vi "Tick Quadrature State.vi"(7 "Forward? (T)":bool=TRUE, 8 "error in (no error)":errorcluster, 9 "Current State":i32, 10 "Channels":string[](array[string])=[" ", ""], 11 "WorkspaceManager in":T1) -> (0 "error out":errorcluster, 1 "New State":i32, 3 "WorkspaceManager out":T1)   [LabVIEW 2026, in "Scan Engine Specialty Digital System Tests.lvclass"]
uses:
  Scan Engine Specialty Digital System Tests.lvclass
  <vilib>/NI/VeriStand Custom Device Testing Tools/VeriStandTestUtilities/VeriStandTestUtilities.lvlib
  <vilib>/NI VeriStand/Execution/Workspace/WorkspaceAPI.ctl
  <vilib>/NI VeriStand/Execution/Workspace/NI_VS Workspace ExecutionAPI.lvlib
  NationalInstruments.VeriStand.ClientAPI
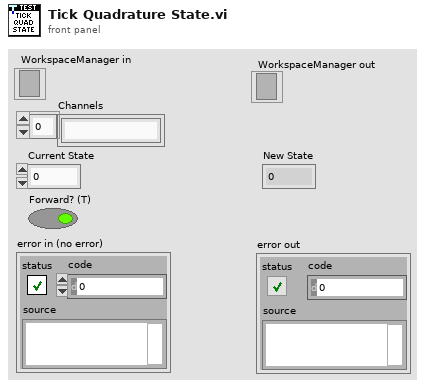
[diagram p1: front panel]
types:
  T1 = typedef "NI_VS Workspace ExecutionAPI.lvlib/WorkspaceAPI.ctl" = refnum<k24>
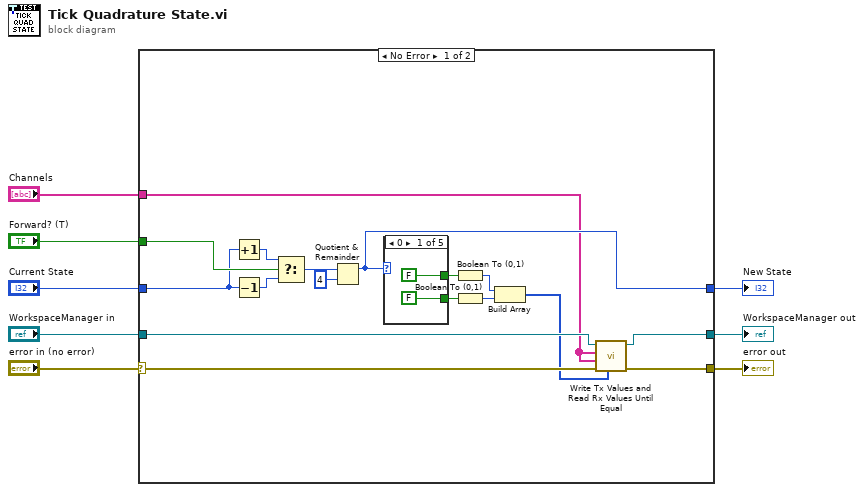
[diagram p0: block diagram]
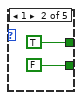
[diagram p2: hidden frame]
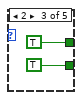
[diagram p3: hidden frame]
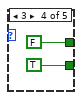
[diagram p4: hidden frame]
diagram:
  n1 = case shown="No Error" "error in (no error)" {
    selector: "error in (no error)" -> [w22 w36]
    tunnel: "Forward? (T)" -> [w25 _]
    tunnel: "WorkspaceManager in" -> [w24 w35]
    tunnel: [w23 w35] -> w6
    tunnel: [w21 w36] -> w4
    tunnel: [w11 w34] -> w1
    tunnel: "Channels" -> [w9 _]
    tunnel: "Current State" -> [w10 w34]
    frame No Error {
      n2 = Increment(x=w10) -> (x+1=w20:i32)
      n3 = Decrement(x=w10) -> (x-1=w19:i32)
      n4 = Select(t=w20, s=w25, f=w19) -> (s? t:f=w18:i32)
      n5 = Quotient & Remainder(x=w18, y=4) -> (x-y*floor(x/y)=w11:i32)  [unwired: 1 out]
      n6 = case shown="0" w11 {
        tunnel: [FALSE TRUE TRUE FALSE _] -> w16
        tunnel: [FALSE FALSE TRUE TRUE _] -> w15
        frame 0 {
        }
        frame 1 {
        }
        frame 2 {
        }
        frame 3 {
        }
        frame Default {
        }
      }
      n7 = Boolean To (0,1)(Boolean=w16) -> (0, 1=w14:i16)
      n8 = Boolean To (0,1)(Boolean=w15) -> (0, 1=w13:i16)
      n9 = Build Array(w14, w13) -> (w12:i16[])
      n10 = call <vilib>:"Write Tx Values and Read Rx Values Until Equal.vi"("Tx values"=w12, "error in"=w22, "Rx aliases"=w9, "Tx aliases"=w9, "workspace manager in"=w24) -> ("error out"=w21:errorcluster, "workspace manager out"=w23:T1)  [unwired: 4 in, 1 out]
    }
    frame Error {
    }
  }
  "WorkspaceManager out" <- w6
  "error out" <- w4
  "New State" <- w1
